vi "Zaber A Series Control Panel.vi"() -> ()   [LabVIEW 2013]
doc: "This VI is a control panel that allows the user to perform a variety of commands and motions, see what devices are connected, read and change settings and track the movements. It is both an example of the way you can use the instrument library as well as a versatile tool for everyday usage."
uses:
  Zaber A Series.lvlib
  <vilib>/Utility/file.llb/Read Delimited Spreadsheet (string).vi
panel:
  out "Motion Type":string[](array[string])
  out "Microstep\nSize":dbl[](array[numeric])
  out "Model Name":string[](array[string])
  out "Device Number\n& Axis":string[](array[string])
  in  "Command List":string(combo)
  in  "Setting":string(combo)
  in  "Data":string
  in  "Units (0: microsteps)":u16(ring) items=["microsteps", "microns", "millimeters", "inches"]
  in  "Movement Type (0: relative)":u16(ring) items=["relative", "absolute"]
  in  "Home":bool
  out "Command Responses":string[](array[string])
  in  "Identify Devices":bool
  in  "Device Number & Axis":string(combo)
  in  "Start Tracking":bool
  out "Position":dbl format="%#_15f"
  out "Current Value":string
  in  "Execute Movement":bool
  in  "Move Distance (0)":dbl format="%#_12f"
  in  "Microstep Size (0)":dbl
  in  "Send Command":bool
  in  "Value to Send":string
  in  "Change Setting":bool
  in  "Get Setting":bool
  in  "VISA resource name":refnum<visa-resource-name>
  in  "Close Port":bool
  in  "Open Port":bool
  in  "Quit":bool
  # "Zaber ASCII Control Panel"
  # "(c) 2017 Zaber Technologies.  ALL RIGHTS RESERVED."
  # "Port Settings"
  # "Shared Settings"
  # "Position Tracking"
  # "Read and Modify Settings"
  # "Send Command"
  # "Identify Connected Devices"
  # "Send Movement"
  # "Home Devices"
  # "See note below."
  # "Identifying device models requires an external lookup\ntable in the form of a .CSV file. A Python script that\ngenerates this file can be found at\nhttp://www.zaber.com/wiki/Software/ASCII_Labview_Driver"
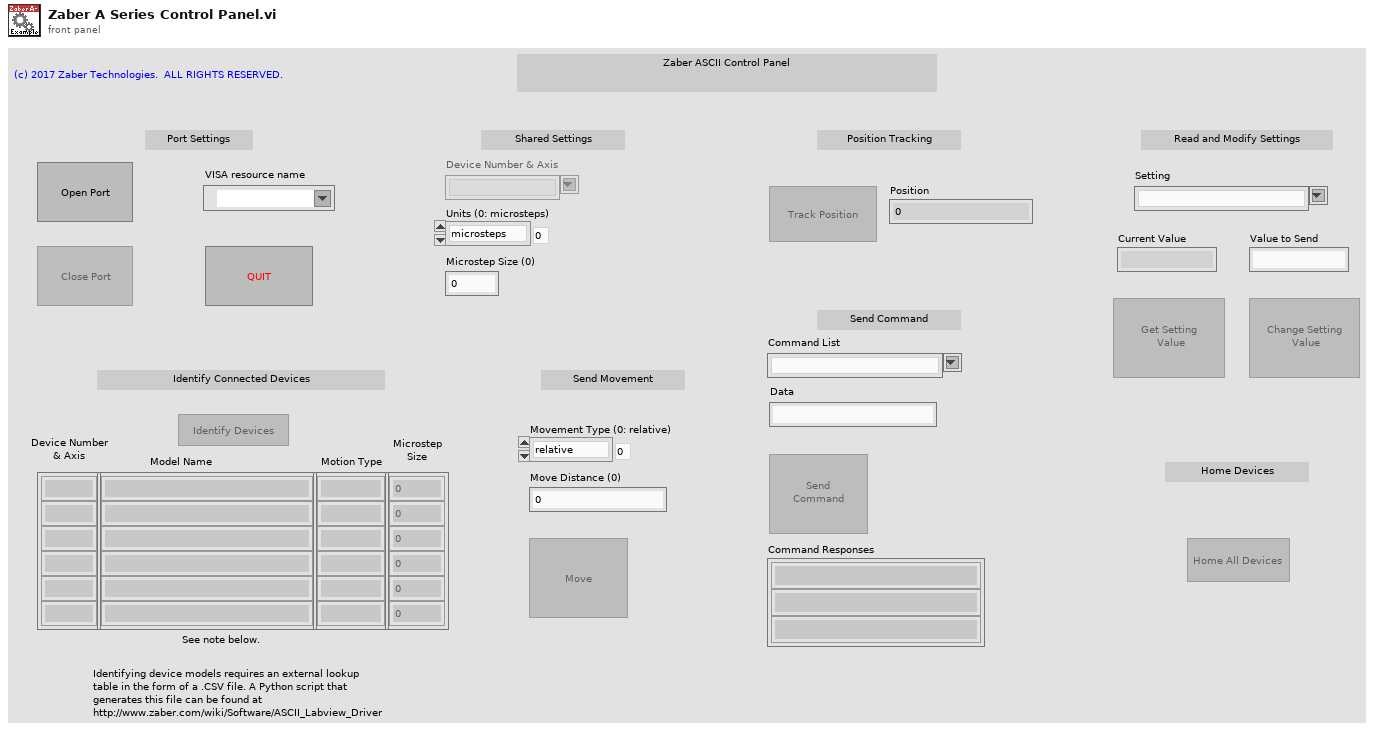
[diagram p1: front panel]
types:
  T1 = enum8{"Enabled", "Disabled", "Disabled and Grayed Out"}
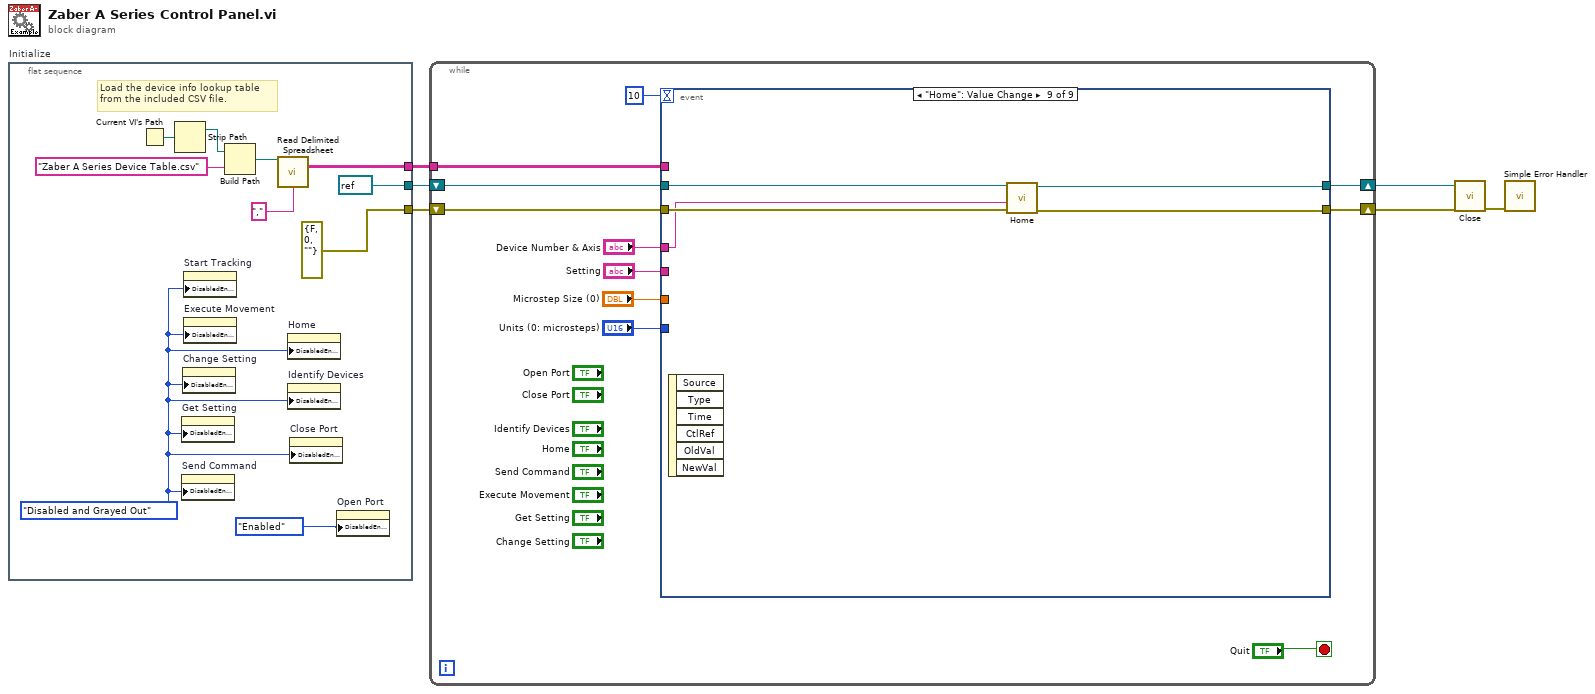
[diagram p0: block diagram]
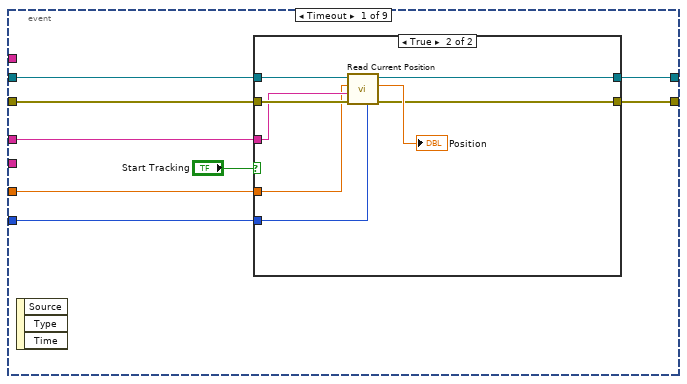
[diagram p2: hidden frame]
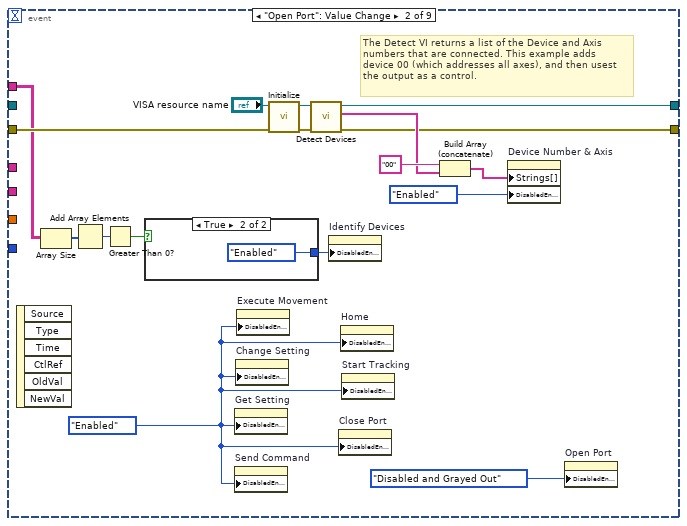
[diagram p4: hidden frame]
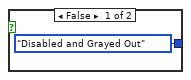
[diagram p5: hidden frame]
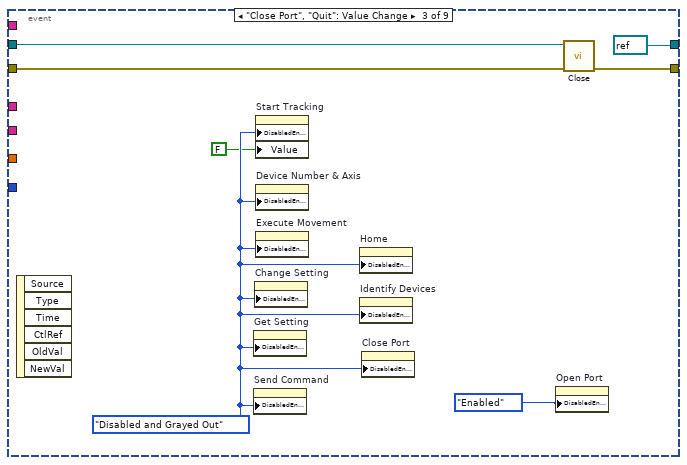
[diagram p6: hidden frame]
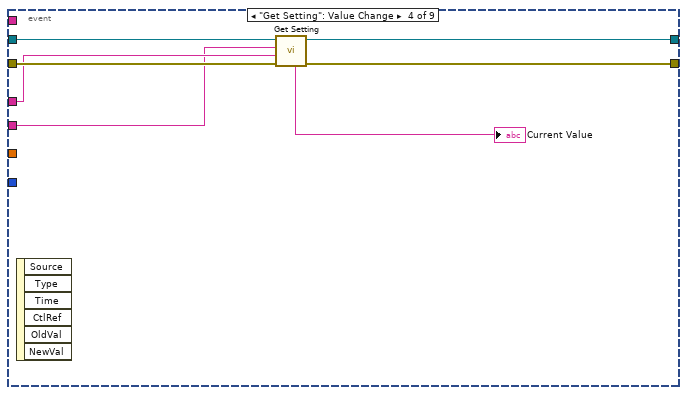
[diagram p7: hidden frame]
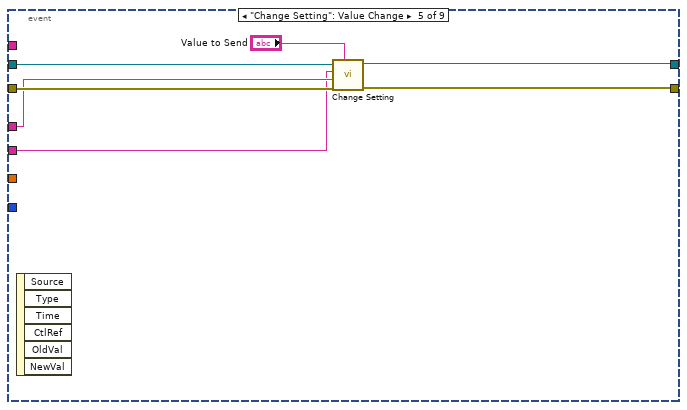
[diagram p8: hidden frame]
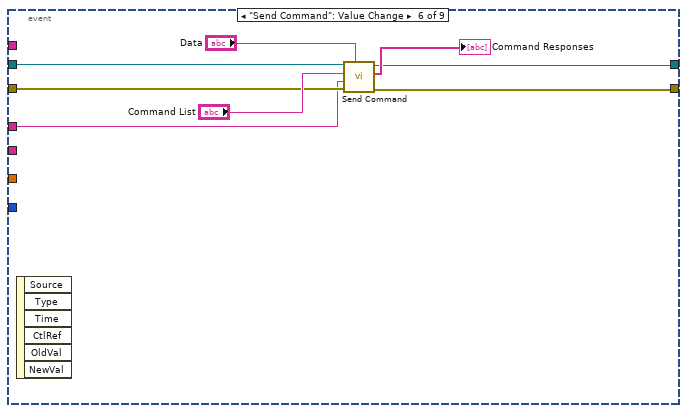
[diagram p9: hidden frame]
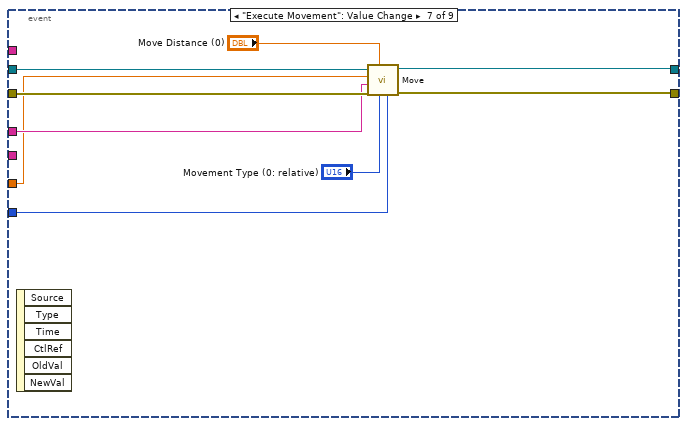
[diagram p10: hidden frame]
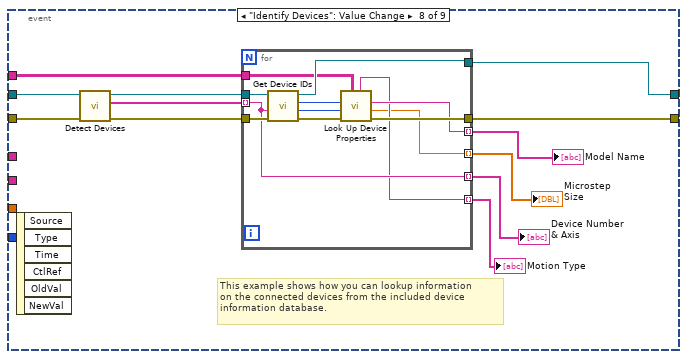
[diagram p11: hidden frame]
diagram:
  n1 = flat-sequence "Initialize" {
    tunnel: [errorcluster {"status"=FALSE, "code"=0, "source"=""} ("error out")] -> w6
    tunnel: [w10] -> w2
    tunnel: [refnum<visa-resource-name> refnum ("VISA resource name")] -> w1
    frame #0 {
      w7 = T1."Disabled and Grayed Out" ("Disabled")
      # "Load the device info lookup table\nfrom the included CSV file."
      n2 = Current VI's Path() -> (path=w14:path)
      n3 = Strip Path(path=w14) -> (stripped path=w15:path)  [unwired: 1 out]
      n4 = property on="Get Setting" class="Bool"("DisabledEnum"=w7) -> ()  [unwired: 2 in, 2 out]
      n5 = property on="Send Command" class="Bool"("DisabledEnum"=w7) -> ()  [unwired: 2 in, 2 out]
      n6 = property on="Change Setting" class="Bool"("DisabledEnum"=w7) -> ()  [unwired: 2 in, 2 out]
      n7 = property on="Start Tracking" class="Bool (strict)"("DisabledEnum"=w7) -> ()  [unwired: 2 in, 2 out]
      n8 = property on="Execute Movement" class="Bool"("DisabledEnum"=w7) -> ()  [unwired: 2 in, 2 out]
      n9 = Build Path(base path=w15, name or relative path="Zaber A Series Device Table.csv") -> (appended path=w12:path)
      n10 = call-poly <vilib>:"Read Delimited Spreadsheet.vi"("file path (dialog if empty)"=w12, "delimiter (\\t)"="," ("delimiter (\\t)")) -> ("all rows"=w10:string[][])  [unwired: 8 in, 5 out]
      n11 = property on="Home" class="Bool"("DisabledEnum"=w7) -> ()  [unwired: 2 in, 2 out]
      n12 = property on="Identify Devices" class="Bool"("DisabledEnum"=w7) -> ()  [unwired: 2 in, 2 out]
      n13 = property on="Close Port" class="Bool"("DisabledEnum"=w7) -> ()  [unwired: 2 in, 2 out]
      n14 = property on="Open Port" class="Bool"("DisabledEnum"=T1."Enabled" ("Disabled")) -> ()  [unwired: 2 in, 2 out]
    }
  }
  n15 = while {
    shift-right: [w23] -> w5
    shift-left: w1 -> [w25]
    shift-right: [w22] -> w4
    shift-left: w6 -> [w24]
    tunnel: w2 -> [w26]
    stop <- "Quit" stop-if-true
    n16 = event shown="[8] \"Home\": Value Change" {
      selector: _ -> [_ _ _ _ _ _ _ _ _]
      dyn-events: _ -> [_ _ _ _ _ _ _ _ _]
      timeout: u32 10 ("milliseconds to wait") -> [_ _ _ _ _ _ _ _ _]
      tunnel: w26 -> [_ w50 _ _ _ _ _ w103 _]
      tunnel: w25 -> [w34 _ w71 w78 w84 w90 w100 w107 w131]
      tunnel: w24 -> [w33 w55 w70 w77 w82 w89 w99 w106 w129]
      tunnel: [w31 w54 w68 w75 w81 w88 w98 w104 w128] -> w22
      tunnel: [w32 w53 refnum<visa-resource-name> refnum ("VISA resource name") w76 w83 w87 w97 w105 w130] -> w23
      tunnel: "Device Number & Axis" -> [w30 _ _ w74 w80 w86 w96 _ w127]
      tunnel: "Setting" -> [_ _ _ w73 w79 _ _ _ _]
      tunnel: "Microstep Size (0)" -> [w29 _ _ _ _ _ w95 _ _]
      tunnel: "Units (0: microsteps)" -> [w28 _ _ _ _ _ w94 _ _]
      event Timeout {
        n17 = event-data() -> ()  [unwired: 1 in, 3 out]
        n18 = case shown="True" "Start Tracking" {
          tunnel: w34 -> [w37 w44]
          tunnel: w33 -> [w36 w42]
          tunnel: [w37 w43] -> w32
          tunnel: [w36 w41] -> w31
          tunnel: w30 -> [_ w40]
          tunnel: w29 -> [_ w39]
          tunnel: w28 -> [_ w38]
          frame False {
          }
          frame True {
            n19 = call "Read Current Position.vi"("Units (0: microsteps)"=w38, "error in (no error)"=w42, "Device and Axis"=w40, "Microstep Size (0)"=w39, "VISA resource name"=w44) -> ("error out"=w41:errorcluster, "Position"=→"Position":dbl, "VISA resource name out"=w43:refnum<visa-resource-name>)  [unwired: 4 in]
          }
        }
      }
      event "Open Port": Value Change {
        w51 = T1."Enabled" ("Disabled")
        # "The Detect VI returns a list of the Device and Axis\nnumbers that are connected. This example adds\ndevice 00 (which addresses all axes), and then usest\nthe output as a control."
        n20 = event-data() -> ()  [unwired: 1 in, 6 out]
        n21 = Array Size(array=w50) -> (size(s)=w49:i32[])
        n22 = Add Array Elements(numeric array=w49) -> (sum=w48:i32)
        n23 = Greater Than 0?(x=w48) -> (x > 0?=w47:bool)
        n24 = case shown="True" w47 {
          tunnel: [T1."Disabled and Grayed Out" ("Disabled") T1."Enabled" ("Disabled")] -> w46
          frame False {
          }
          frame True {
          }
        }
        n25 = property on="Get Setting" class="Bool"("DisabledEnum"=w51) -> ()  [unwired: 2 in, 2 out]
        n26 = property on="Send Command" class="Bool"("DisabledEnum"=w51) -> ()  [unwired: 2 in, 2 out]
        n27 = property on="Change Setting" class="Bool"("DisabledEnum"=w51) -> ()  [unwired: 2 in, 2 out]
        n28 = property on="Execute Movement" class="Bool"("DisabledEnum"=w51) -> ()  [unwired: 2 in, 2 out]
        n29 = call "Initialize.vi"("error in (no error)"=w55, "VISA resource name"="VISA resource name") -> ("error out"=w58:errorcluster, "VISA resource name out"=w57:refnum<visa-resource-name>)  [unwired: 8 in]
        n30 = call "Detect Devices.vi"("error in (no error)"=w58, "VISA resource name"=w57) -> ("error out"=w54:errorcluster, "Connected Devices and Axes"=w60:string[], "VISA resource name out"=w53:refnum<visa-resource-name>)  [unwired: 6 in, 1 out]
        n31 = property on="Identify Devices" class="Bool"("DisabledEnum"=w46) -> ()  [unwired: 2 in, 2 out]
        n32 = property on="Close Port" class="Bool"("DisabledEnum"=w51) -> ()  [unwired: 2 in, 2 out]
        n33 = property on="Home" class="Bool"("DisabledEnum"=w51) -> ()  [unwired: 2 in, 2 out]
        n34 = property on="Start Tracking" class="Bool (strict)"("DisabledEnum"=w51) -> ()  [unwired: 2 in, 2 out]
        n35 = Build Array (concatenate)("00", w60) -> (w61:string[])
        n36 = property on="Device Number & Axis" class="CmbBox"("Strings[]"=w61, "DisabledEnum"=T1."Enabled" ("Disabled")) -> ()  [unwired: 2 in, 2 out]
        n37 = property on="Open Port" class="Bool"("DisabledEnum"=T1."Disabled and Grayed Out" ("Disabled")) -> ()  [unwired: 2 in, 2 out]
      }
      event "Close Port", "Quit": Value Change {
        w66 = T1."Disabled and Grayed Out" ("Disabled")
        n38 = event-data() -> ()  [unwired: 1 in, 6 out]
        n39 = property on="Get Setting" class="Bool"("DisabledEnum"=w66) -> ()  [unwired: 2 in, 2 out]
        n40 = property on="Send Command" class="Bool"("DisabledEnum"=w66) -> ()  [unwired: 2 in, 2 out]
        n41 = property on="Change Setting" class="Bool"("DisabledEnum"=w66) -> ()  [unwired: 2 in, 2 out]
        n42 = property on="Start Tracking" class="Bool (strict)"("DisabledEnum"=w66, "Value"=FALSE ("Start Tracking")) -> ()  [unwired: 2 in, 2 out]
        n43 = property on="Device Number & Axis" class="CmbBox"("DisabledEnum"=w66) -> ()  [unwired: 2 in, 2 out]
        n44 = property on="Execute Movement" class="Bool"("DisabledEnum"=w66) -> ()  [unwired: 2 in, 2 out]
        n45 = property on="Home" class="Bool"("DisabledEnum"=w66) -> ()  [unwired: 2 in, 2 out]
        n46 = property on="Identify Devices" class="Bool"("DisabledEnum"=w66) -> ()  [unwired: 2 in, 2 out]
        n47 = property on="Close Port" class="Bool"("DisabledEnum"=w66) -> ()  [unwired: 2 in, 2 out]
        n48 = property on="Open Port" class="Bool"("DisabledEnum"=T1."Enabled" ("Disabled")) -> ()  [unwired: 2 in, 2 out]
        n49 = call "Close.vi"("error in (no error)"=w70, "VISA resource name"=w71) -> ("error out"=w68:errorcluster)  [unwired: 9 in]
      }
      event "Get Setting": Value Change {
        n50 = event-data() -> ()  [unwired: 1 in, 6 out]
        n51 = call "Get Setting.vi"("error in (no error)"=w77, "Device and Axis"=w74, "Setting"=w73, "VISA resource name"=w78) -> ("error out"=w75:errorcluster, "VISA resource name out"=w76:refnum<visa-resource-name>, "First Response Data"=→"Current Value":string)  [unwired: 2 in, 3 out]
      }
      event "Change Setting": Value Change {
        n52 = event-data() -> ()  [unwired: 1 in, 6 out]
        n53 = call "Change Setting.vi"("Data"="Value to Send", "error in (no error)"=w82, "Device and Axis"=w80, "Setting"=w79, "VISA resource name"=w84) -> ("error out"=w81:errorcluster, "VISA resource name out"=w83:refnum<visa-resource-name>)  [unwired: 5 in]
      }
      event "Send Command": Value Change {
        n54 = event-data() -> ()  [unwired: 1 in, 6 out]
        n55 = call "Send Command.vi"("Data"="Data", "error in (no error)"=w89, "Device and Axis"=w86, "Command"="Command List", "VISA resource name"=w90) -> ("error out"=w88:errorcluster, "Response String Array"=→"Command Responses":string[], "VISA resource name out"=w87:refnum<visa-resource-name>)  [unwired: 1 in, 3 out]
      }
      event "Execute Movement": Value Change {
        n56 = event-data() -> ()  [unwired: 1 in, 6 out]
        n57 = call "Move.vi"("Units (0: microsteps)"=w94, "Movement Type (0: relative)"="Movement Type (0: relative)", "Move Distance (0)"="Move Distance (0)", "error in (no error)"=w99, "Device and Axis"=w96, "Microstep Size (0)"=w95, "VISA resource name"=w100) -> ("error out"=w98:errorcluster, "VISA resource name out"=w97:refnum<visa-resource-name>)  [unwired: 3 in]
      }
      event "Identify Devices": Value Change {
        # "This example shows how you can lookup information\non the connected devices from the included device \ninformation database."
        n58 = event-data() -> ()  [unwired: 1 in, 6 out]
        n59 = call "Detect Devices.vi"("error in (no error)"=w106, "VISA resource name"=w107) -> ("error out"=w109:errorcluster, "Connected Devices and Axes"=w110:string[], "VISA resource name out"=w108:refnum<visa-resource-name>)  [unwired: 6 in, 1 out]
        n60 = for {
          tunnel: w108 -> [w126]
          tunnel: w109 -> [w125]
          tunnel: [w121] -> w104
          tunnel: w110 -> [w120] mode=indexing
          tunnel: [w120] -> w111 mode=indexing
          tunnel: [w119] -> w112 mode=indexing
          tunnel: [w115] -> w113 mode=indexing
          tunnel: [w118] -> w114 mode=indexing
          tunnel: [w117] -> w105
          tunnel: w103 -> [w116]
          n61 = call "Get Device IDs.vi"("error in (no error)"=w125, "Device and Axis"=w120, "VISA resource name"=w126) -> ("error out"=w122:errorcluster, "Peripheral ID"=w123:i32, "Device ID"=w124:i32, "VISA resource name out"=w117:refnum<visa-resource-name>)  [unwired: 5 in]
          n62 = call "Look Up Device Properties.vi"("Lookup Table"=w116, "error in (no error)"=w122, "Peripheral ID (0)"=w123, "Device ID"=w124) -> ("error out"=w121:errorcluster, "Microstep Size"=w115:dbl, "Device Name"=w119:string, "Motion Type"=w118:string)  [unwired: 4 in]
        }
        "Device Number\n& Axis" <- w111
        "Model Name" <- w112
        "Microstep\nSize" <- w113
        "Motion Type" <- w114
      }
      event "Home": Value Change {
        n63 = event-data() -> ()  [unwired: 1 in, 6 out]
        n64 = call "Home.vi"("error in (no error)"=w129, "Device and Axis"=w127, "VISA resource name"=w131) -> ("error out"=w128:errorcluster, "VISA resource name out"=w130:refnum<visa-resource-name>)  [unwired: 7 in]
      }
    }
  }
  n65 = call "Close.vi"("error in (no error)"=w4, "VISA resource name"=w5) -> ("error out"=w3:errorcluster)  [unwired: 9 in]
  n66 = call <vilib>:"Simple Error Handler.vi"("error in (no error)"=w3) -> ()  [unwired: 4 in, 5 out]
